vi "Run.vi"(9 "Team In":refnum<class "Team.lvclass">, 11 "MySquare in":refnum<class "MySquare.lvclass">) -> (1 "Team":refnum<class "Team.lvclass">, 2 "Run Result":T1, 3 "MySquare out":refnum<class "MySquare.lvclass">)   [LabVIEW 2020, in "Clones.lvlib" / "MySquare.lvclass"]
doc: "This VI is called on every active square each turn of the game for the square to decide what action to take."
uses:
  MySquare.lvclass
  SquareBattle/Run Result.ctl
  SquareBattle/Square/Square.lvclass
  SquareBattle/Action.ctl
  SquareBattle/Direction.ctl
  SquareBattle/Team/Team.lvclass
  MyTeam/MyTeam.lvclass
  C:/dev/sol-squarebattle/SquareBattle/Team/Team.lvclass
  MySquare.lvclass/MySquare.ctl
  SquareBattle/SquareBattle.lvlib
  C:/dev/sol-squarebattle/SquareBattle/Square/Square.lvclass
  C:/dev/sol-squarebattle/Squares/Clones/SquareTeam/MySquare/MySquare.lvclass
  C:/dev/sol-squarebattle/Squares/Clones/SquareTeam/MyTeam/MyTeam.lvclass
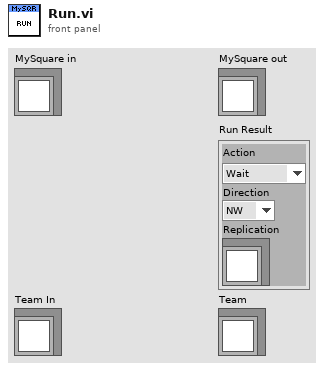
[diagram p1: front panel]
types:
  T1 = typedef "SquareBattle.lvlib/Run Result.ctl" = cluster{"Action":T2, "Direction":T3, "Replication":refnum<class "Square.lvclass">}
  T2 = typedef "SquareBattle.lvlib/Action.ctl" = enum16{"Wait", "Move", "Attack", "Replicate"}
  T3 = typedef "SquareBattle.lvlib/Direction.ctl" = enum16{"NW", "N", "NE", "E", "SE", "S", "SW", "W"}
  T4 = enum16{"NW", "N", "NE", "E", "SE", "S", "SW", "W"}
  T5 = typedef "SquareBattle.lvlib/Location Status.ctl" = cluster{"Empty":bool, "Friend":bool, "Enemy":bool}
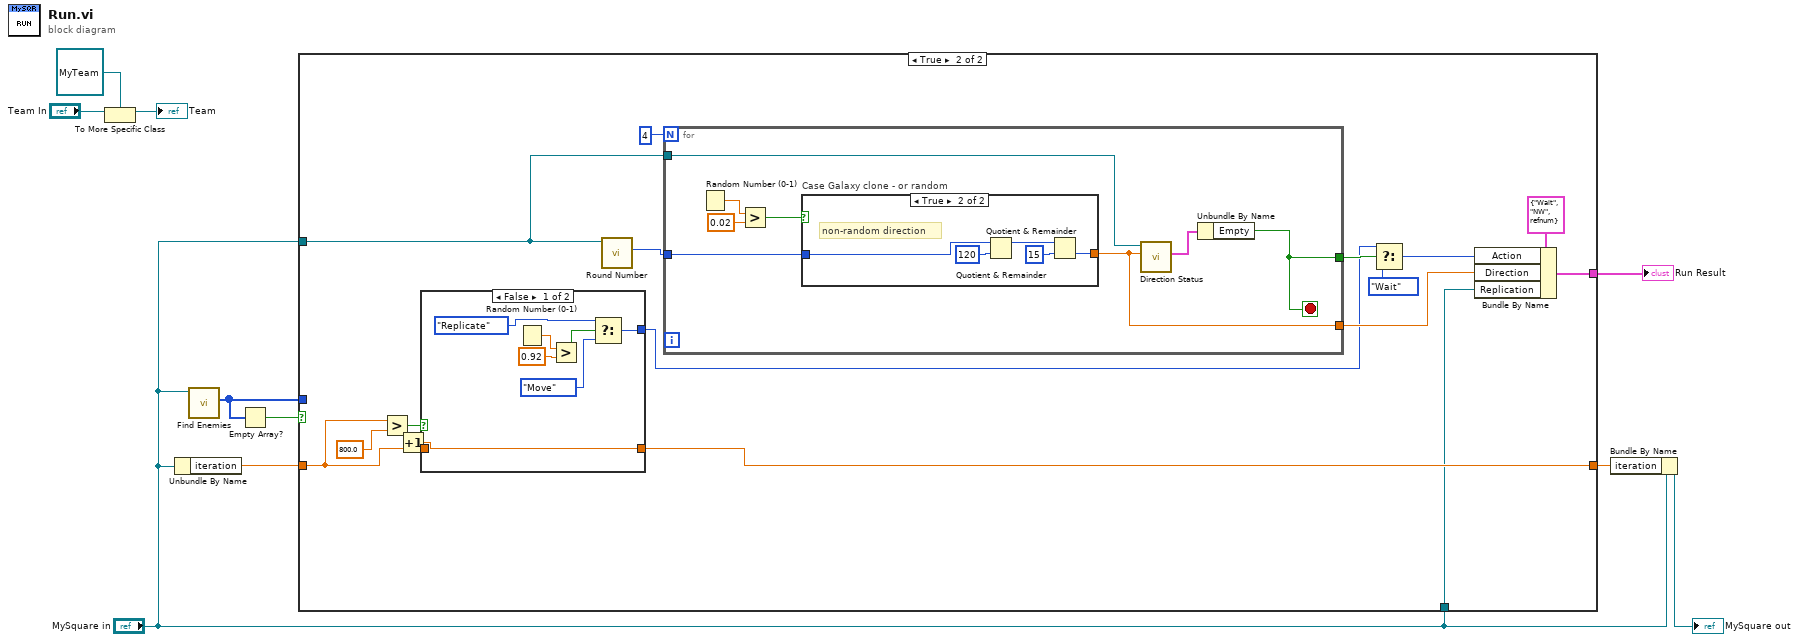
[diagram p0: block diagram]
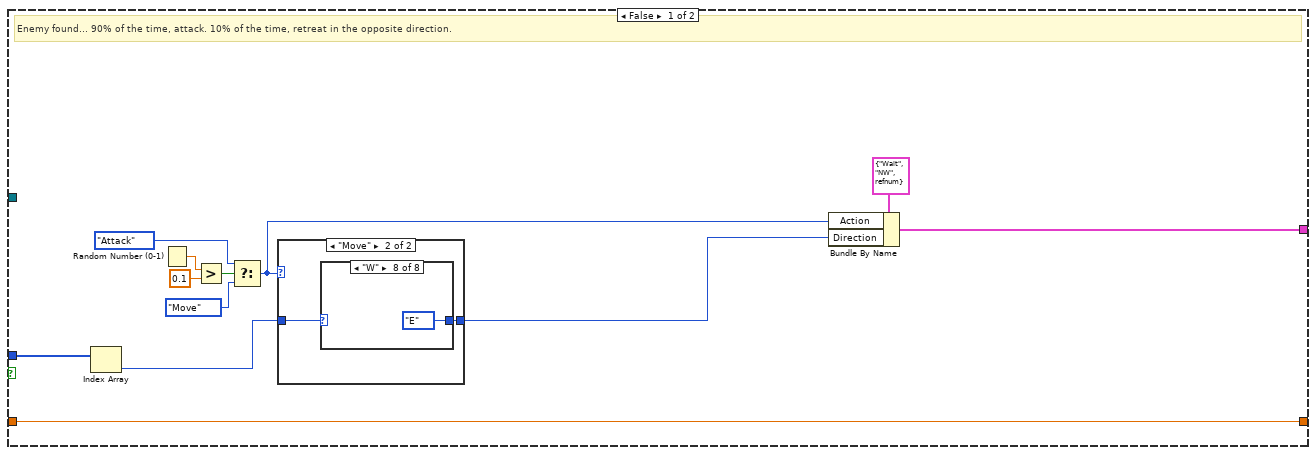
[diagram p2: hidden frame]
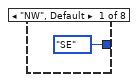
[diagram p4: hidden frame]
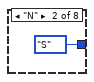
[diagram p5: hidden frame]
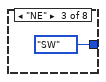
[diagram p6: hidden frame]
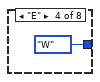
[diagram p7: hidden frame]
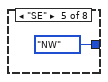
[diagram p8: hidden frame]
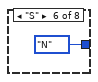
[diagram p9: hidden frame]
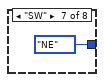
[diagram p10: hidden frame]
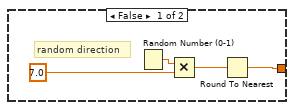
[diagram p11: hidden frame]
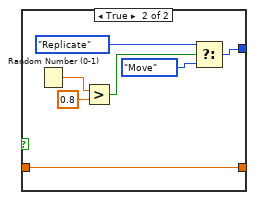
[diagram p12: hidden frame]
diagram:
  n1 = To More Specific Class(target class=refnum<class "MyTeam.lvclass"> refnum ("SquareTeam.lvlib:MyTeam.lvclass"), reference="Team In") -> (specific class reference=→"Team":refnum<class "MyTeam.lvclass">)  [unwired: 1 in, 1 out]
  n2 = Unbundle By Name("MySquare in") -> ("iteration"=w3:dbl)
  n3 = call "Find Enemies.vi"("Square in"="MySquare in") -> ("Enemy Directions"=w5:T3[])  [unwired: 9 in, 1 out]
  n4 = Empty Array?(array=w5) -> (empty?=w6:bool)
  n5 = case shown="True" w6 {
    tunnel: w5 -> [w14 _]
    tunnel: [w22 w45] -> w4
    tunnel: w3 -> [w22 w46]
    tunnel: [w11 w39] -> w2
    tunnel: "MySquare in" -> [_ w42]
    tunnel: "MySquare in" -> [_ w40]
    frame False {
      # "Enemy found... 90% of the time, attack. 10% of the time, retreat in the opposite direction."
      n6 = Index Array(array=w14) -> (element=w13:T3)  [unwired: 1 in]
      n7 = Random Number (0-1)() -> (number: 0 to 1=w21:dbl)
      n8 = Greater?(x=w21, y=0.1) -> (0:w19:bool)
      n9 = Select(t=enum16{"Wait", "Move", "Attack", "Replicate"}."Attack" ("Action"), s=w19, f=enum16{"Wait", "Move", "Attack", "Replicate"}."Move" ("Action")) -> (s? t:f=w15:enum16{"Wait", "Move", "Attack", "Replicate"})
      n10 = case shown="\"Move\"" w15 {
        tunnel: w13 -> [w23 w25]
        tunnel: [w23 w24] -> w12
        frame "Attack", Default {
        }
        frame "Move" {
          n11 = case shown="\"W\"" w25 {
            tunnel: [T4."SE" ("Direction 2") T4."S" ("Direction 2") T4."SW" ("Direction 2") T4."W" ("Direction 2") T4."NW" ("Direction 2") T4."N" ("Direction 2") T4."NE" ("Direction 2") T4."E" ("Direction 2")] -> w24
            frame "NW", Default {
            }
            frame "N" {
            }
            frame "NE" {
            }
            frame "E" {
            }
            frame "SE" {
            }
            frame "S" {
            }
            frame "SW" {
            }
            frame "W" {
            }
          }
        }
      }
      n12 = Bundle By Name(cluster=T1 {"Action"=enum."Wait", "Direction"=enum."NW", "Replication"=refnum} ("Run Result"), "Action"=w15, "Direction"=w12) -> (w11:T1)
    }
    frame True {
      n13 = Greater?(x=w46, y=800.0) -> (0:w47:bool)
      n14 = case shown="False" w47 {
        tunnel: w46 -> [w72 w79]
        tunnel: [w73 w80] -> w34
        tunnel: [w71 w79] -> w45
        frame False {
          n15 = Increment(x=w72) -> (x+1=w71:dbl)
          n16 = Random Number (0-1)() -> (number: 0 to 1=w70:dbl)
          n17 = Greater?(x=w70, y=0.92) -> (0:w68:bool)
          n18 = Select(t=enum16{"Wait", "Move", "Attack", "Replicate"}."Replicate" ("Action"), s=w68, f=enum16{"Wait", "Move", "Attack", "Replicate"}."Move" ("Action")) -> (s? t:f=w73:enum16{"Wait", "Move", "Attack", "Replicate"})
        }
        frame True {
          n19 = Random Number (0-1)() -> (number: 0 to 1=w78:dbl)
          n20 = Greater?(x=w78, y=0.8) -> (0:w76:bool)
          n21 = Select(t=enum16{"Wait", "Move", "Attack", "Replicate"}."Replicate" ("Action"), s=w76, f=enum16{"Wait", "Move", "Attack", "Replicate"}."Move" ("Action")) -> (s? t:f=w80:enum16{"Wait", "Move", "Attack", "Replicate"})
        }
      }
      n22 = call "Round Number.vi"("Square in"=w42) -> ("Round Number"=w43:u32)  [unwired: 8 in, 2 out]
      n23 = for {
        N: 4 -> [_]
        tunnel: w43 -> [w56]
        tunnel: [w49] -> w35
        tunnel: w42 -> [w52]
        tunnel: [w50] -> w38
        stop <- w50 stop-if-true
        n24 = Random Number (0-1)() -> (number: 0 to 1=w54:dbl)
        n25 = Greater?(x=w54, y=0.02) -> (0:w55:bool)
        n26 = case "Case Galaxy clone - or random" shown="True" w55 {
          tunnel: w56 -> [_ w65]
          tunnel: [w57 w64] -> w49
          frame False {
            # "random direction"
            n27 = Random Number (0-1)() -> (number: 0 to 1=w60:dbl)
            n28 = Multiply(x=w60, y=7.0) -> (x*y=w58:dbl)
            n29 = Round To Nearest(number=w58) -> (nearest integer value=w57:dbl)
          }
          frame True {
            # "non-random direction"
            n30 = Quotient & Remainder(x=w65, y=120) -> (x-y*floor(x/y)=w61:u32)  [unwired: 1 out]
            n31 = Quotient & Remainder(x=w61, y=15) -> (floor(x/y)=w64:u32)  [unwired: 1 out]
          }
        }
        n32 = call "Direction Status.vi"("Direction"=w49, "Square in"=w52) -> ("Status"=w51:T5)  [unwired: 8 in, 1 out]
        n33 = Unbundle By Name(w51) -> ("Empty"=w50:bool)
      }
      n34 = Select(t=w34, s=w38, f=enum16{"Wait", "Move", "Attack", "Replicate"}."Wait" ("Action")) -> (s? t:f=w36:enum16{"Wait", "Move", "Attack", "Replicate"})
      n35 = Bundle By Name(cluster=T1 {"Action"=enum."Wait", "Direction"=enum."NW", "Replication"=refnum} ("Run Result"), "Action"=w36, "Direction"=w35, "Replication"=w40) -> (w39:T1)
    }
  }
  "Run Result" <- w2
  n36 = Bundle By Name(cluster="MySquare in", "iteration"=w4) -> (→"MySquare out":refnum<class "MySquare.lvclass">)
